vi "ServoPickup.vi"   [LabVIEW 2017]
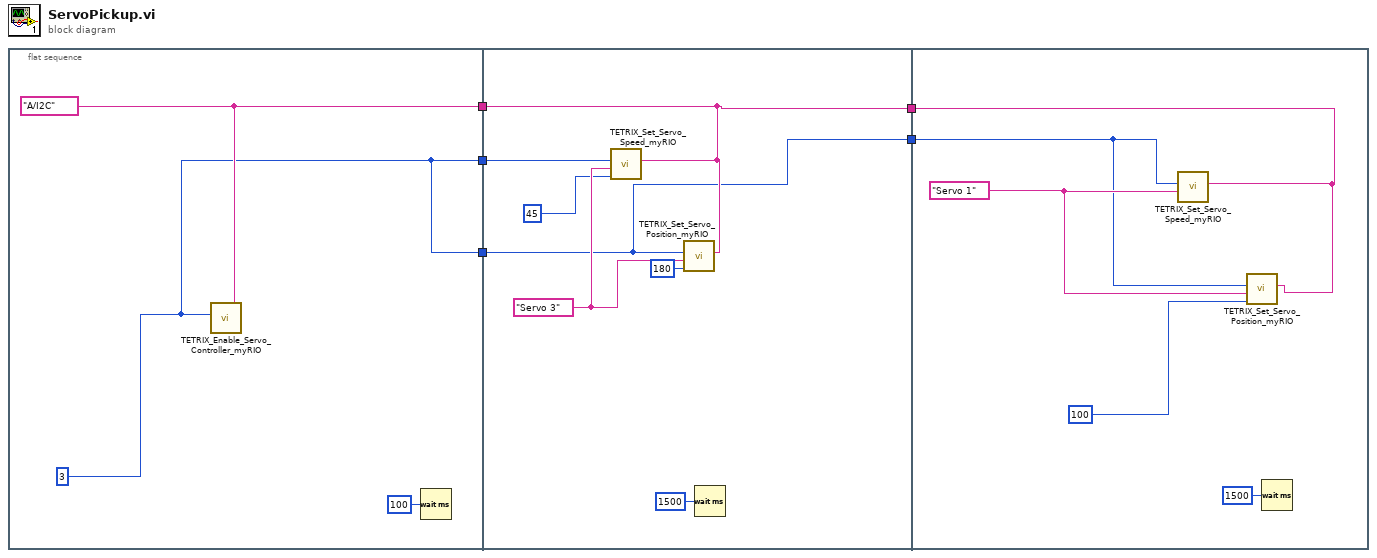
[diagram p0: block diagram]
diagram:
  n1 = flat-sequence {
    tunnel: [w7] -> w5
    tunnel: [w6] -> w4
    tunnel: [w6] -> w3
    tunnel: w5 -> [w10]
    tunnel: w4 -> [w15]
    tunnel: w3 -> [w9]
    tunnel: [w10] -> w2
    tunnel: [w9] -> w1
    tunnel: w2 -> [w20]
    tunnel: w1 -> [w17]
    frame #0 {
      w6 = u8 3 ("Controller ID#  (I2C Address)")
      w7 = tag "A/I2C" ("myRIO MXP Port A/B")
      n2 = call <vilib>:"TETRIX_Enable_Servo_Controller_myRIO.vi"("myRIO MXP Port A/B"=w7, "Controller ID#  (I2C Address)"=w6) -> ()  [unwired: 5 in, 1 out]
      n3 = Wait (ms)(milliseconds to wait=u32 100) -> ()  [unwired: 1 out]
    }
    frame #1 {
      w14 = "Servo 3" ("Select Channel")
      n4 = call <vilib>:"TETRIX_Set_Servo_Speed_myRIO.vi"("myRIO MXP Port A/B"=w10, "Set Servo Speed (0 - 100 percent)"=u8 45, "Select Channel"=w14, "Controller ID#  (I2C Address)"=w15) -> ()  [unwired: 3 in, 1 out]
      n5 = call <vilib>:"TETRIX_Set_Servo_Position_myRIO.vi"("myRIO MXP Port A/B"=w10, "Set Servo Position (0 - 180 degrees)"=u8 180, "Select Channel"=w14, "Controller ID#  (I2C Address)"=w9) -> ()  [unwired: 3 in, 1 out]
      n6 = Wait (ms)(milliseconds to wait=u32 1500) -> ()  [unwired: 1 out]
    }
    frame #2 {
      w19 = "Servo 1" ("Select Channel")
      n7 = call <vilib>:"TETRIX_Set_Servo_Speed_myRIO.vi"("myRIO MXP Port A/B"=w20, "Select Channel"=w19, "Controller ID#  (I2C Address)"=w17) -> ()  [unwired: 4 in, 1 out]
      n8 = call <vilib>:"TETRIX_Set_Servo_Position_myRIO.vi"("myRIO MXP Port A/B"=w20, "Set Servo Position (0 - 180 degrees)"=u8 100, "Select Channel"=w19, "Controller ID#  (I2C Address)"=w17) -> ()  [unwired: 3 in, 1 out]
      n9 = Wait (ms)(milliseconds to wait=u32 1500) -> ()  [unwired: 1 out]
    }
  }
